vi "init_RF_generators.vi"(8 "error in":errorcluster, 11 "HP83623A Generator Settings Array":T1) -> (0 "error out":errorcluster)   [LabVIEW 2013]
uses:
  HP83623A_RF_Generator/HP83623A_array.ctl
  HP83623A_RF_Generator/HP83623A.ctl
  HP83623A_RF_Generator/HP83623A_RF_Generator.lvclass
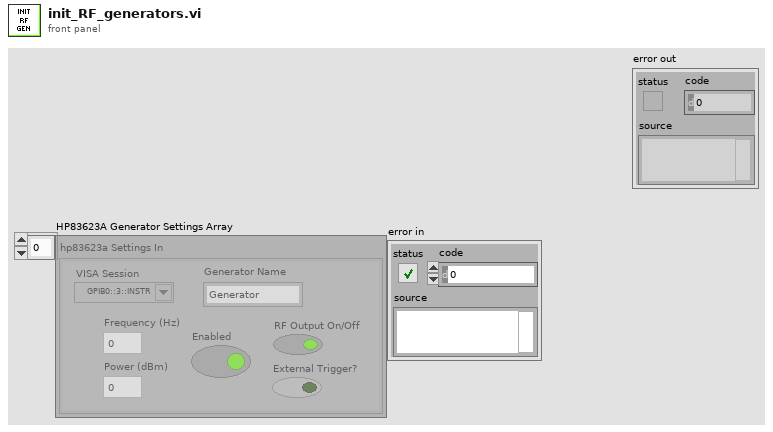
[diagram p1: front panel]
types:
  T1 = typedef "HP83623A_RF_Generator.lvclass/HP83623A_array.ctl" = T2[]
  T2 = typedef "HP83623A_RF_Generator.lvclass/HP83623A.ctl" = cluster{"Frequency (Hz)":dbl, "Power (dBm)":dbl, "Enabled":bool, "initialized":bool, "RF Output On/Off":bool, "External Trigger?":bool, "VISA Session":refnum<visa-resource-name>, "Generator Name":string}
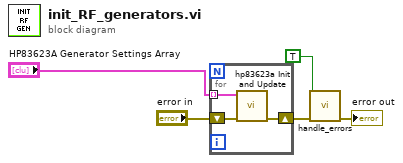
[diagram p0: block diagram]
diagram:
  n1 = for {
    shift-right: [w7] -> w3
    shift-left: "error in" -> [w8]
    tunnel: "HP83623A Generator Settings Array" -> [w6] mode=indexing
    n2 = call "hp83623a Init and Update.vi"("error in (no error)"=w8, "hp83623a Settings (in)"=w6) -> ("error out"=w7:errorcluster)  [unwired: 8 in, 1 out]
  }
  n3 = call "handle_errors.vi"("Exit Operation"=TRUE, "error in (no error)"=w3) -> ("error out"=→"error out":errorcluster)  [unwired: 13 in]
